vi "Simple Move.vi"(8 "error in (no error)":errorcluster, 10 "Move Data cluster":T1, 11 "Motions in":refnum<class "Motions.lvclass">) -> (0 "error out":errorcluster, 3 "Motions out":refnum<class "Motions.lvclass">)   [LabVIEW 2016, in "Hardware.lvlib" / "Motions.lvlib" / "Motions.lvclass"]
uses:
  <userlib>/Common Components/Hardware/Abstract System/Motions/Motions/Motions.lvclass
  <userlib>/Common Components/Hardware/Abstract System/Motions/Motions/Data_Move.ctl
  <userlib>/Common Components/Hardware/Abstract System/Motions/Motions/Motions.lvclass/Motions.ctl
  <userlib>/Common Components/Hardware/Motor/Motor/Motor.lvclass
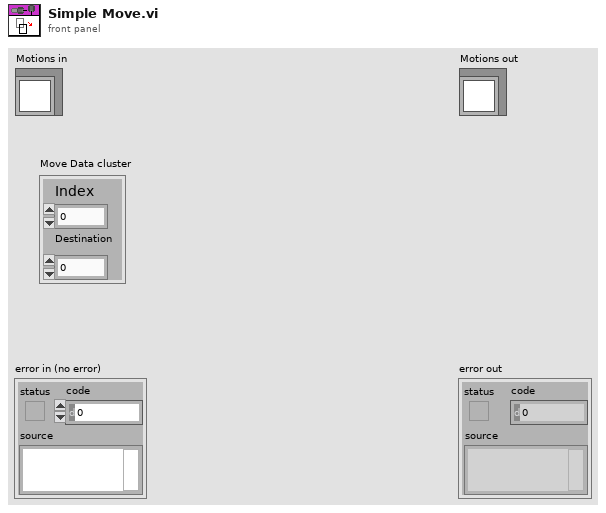
[diagram p1: front panel]
types:
  T1 = typedef "Hardware.lvlib/Motions.lvlib/Motions.lvclass/Data_Move.ctl" = cluster{"Index":i32, "Destination":dbl}
  T2 = typedef "Hardware.lvlib/Motions.lvlib/Motions.lvclass/Motor States.ctl" = cluster{"Connected":bool, "Enabled":bool, "Moving Status":bool, "Soft Moving Status":bool, "Current Pos":dbl, "Target Pos":dbl, "Moving Dir (-1, 0, 1)":i32, "Error Status":bool, "Hard Limit+":bool, "Hard Limit-":bool, "Soft Limit+":bool, "Soft Limit-":bool, "History Dst Stack":refnum<queue>, "Motion Status":bool, "Motion TriggerAction Obj":refnum<class "TriggerAction Q.lvclass">}
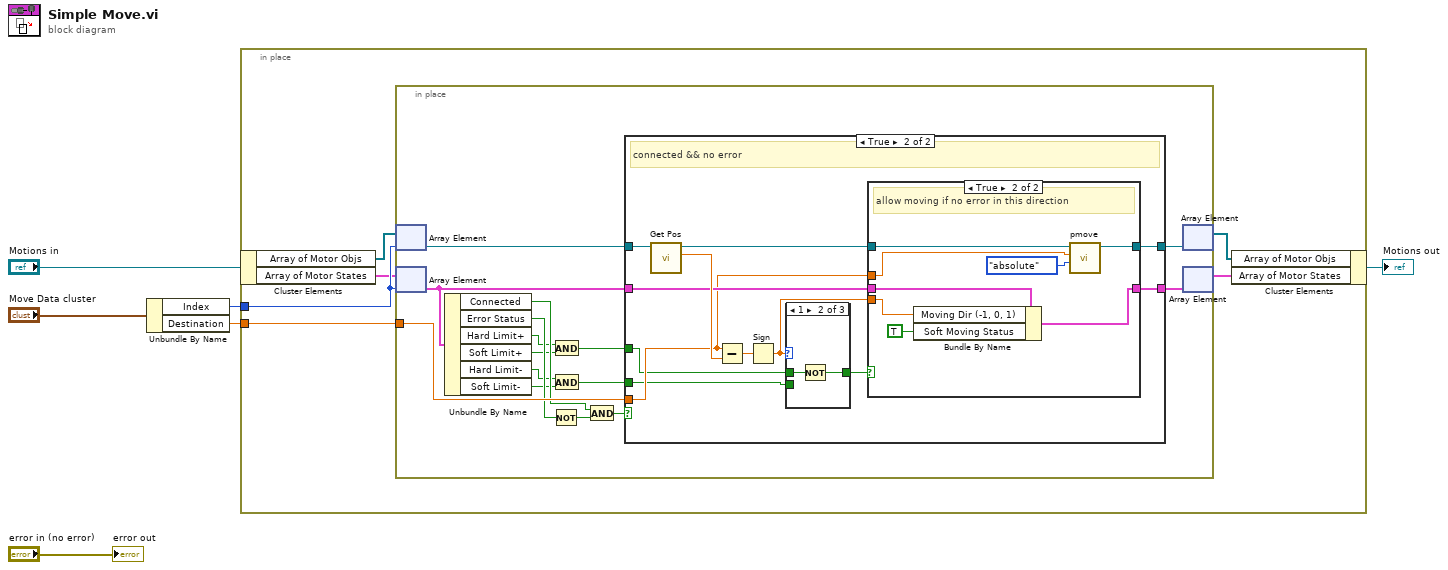
[diagram p0: block diagram]
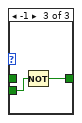
[diagram p4: hidden frame]
diagram:
  n1 = Unbundle By Name("Move Data cluster") -> ("Index"=w2:i32, "Destination"=w1:dbl)
  n2 = in-place {
    in-place-border: w2 -> [w9]
    in-place-border: w1 -> [w10]
    n3 = in-place-cluster #1("Motions in") -> ("Array of Motor Objs"=w12:refnum<class "Motor.lvclass">[], "Array of Motor States"=w8:T2[])
    n4 = in-place {
      in-place-border: w10 -> [w26]
      n5 = in-place-array #2(w12, w9) -> (w27:refnum<class "Motor.lvclass">)
      n6 = in-place-array #3(w8, w9) -> (w25:T2)
      n7 = Unbundle By Name(w25) -> ("Connected"=w23:bool, "Error Status"=w22:bool, "Hard Limit+"=w18:bool, "Soft Limit+"=w17:bool, "Hard Limit-"=w16:bool, "Soft Limit-"=w15:bool)
      n8 = Not(x=w22) -> (.not. x?=w21:bool)
      n9 = And(x=w18, y=w17) -> (x .and. y?=w14:bool)
      n10 = And(x=w16, y=w15) -> (x .and. y?=w13:bool)
      n11 = And(x=w23, y=w21) -> (x .and. y?=w20:bool)
      n12 = case shown="True" w20 {
        tunnel: w27 -> [w28 w34]
        tunnel: w26 -> [_ w35]
        tunnel: w25 -> [w29 w39]
        tunnel: [w29 w38] -> w24
        tunnel: [w28 w36] -> w19
        tunnel: w14 -> [_ w31]
        tunnel: w13 -> [_ w30]
        frame False {
        }
        frame True {
          # "connected && no error"
          n13 = call <userlib>:"Get Pos.vi"("Motor in"=w34) -> ("Position in unit mode (backend)"=w40:dbl, "Motor out"=w37:refnum<class "Motor.lvclass">)  [unwired: 7 in, 2 out]
          n14 = Subtract(x=w35, y=w40) -> (x-y=w41:dbl)
          n15 = Sign(1:w41) -> (0:w33:dbl)
          n16 = case shown="1" w33 {
            tunnel: [_ w42 w44] -> w32
            tunnel: w31 -> [_ w43 _]
            tunnel: w30 -> [_ _ w45]
            frame 0, Default {
            }
            frame 1 {
              n17 = Not(x=w43) -> (.not. x?=w42:bool)
            }
            frame -1 {
              n18 = Not(x=w45) -> (.not. x?=w44:bool)
            }
          }
          n19 = case shown="True" w32 {
            tunnel: w33 -> [_ w55]
            tunnel: w39 -> [w46 w54]
            tunnel: [w46 w53] -> w38
            tunnel: w37 -> [w47 w52]
            tunnel: [w47 w51] -> w36
            tunnel: w35 -> [_ w49]
            frame False {
            }
            frame True {
              # "allow moving if no error in this direction"
              n20 = Bundle By Name(cluster=w54, "Moving Dir (-1, 0, 1)"=w55, "Soft Moving Status"=TRUE) -> (w53:T2)
              n21 = call <userlib>:"pmove.vi"("mode (0: rel; 1: abs)"=enum16{"relative", "absolute"}."absolute", "distance in unit mode"=w49, "Motor in"=w52) -> ("Motor out"=w51:refnum<class "Motor.lvclass">)  [unwired: 7 in, 1 out]
            }
          }
        }
      }
      n22 = in-place-array #2(w19) -> (w11:refnum<class "Motor.lvclass">[])  [unwired: 1 out]
      n23 = in-place-array #3(w24) -> (w7:T2[])  [unwired: 1 out]
    }
    n24 = in-place-cluster #1("Array of Motor Objs"=w11, "Array of Motor States"=w7) -> (→"Motions out":refnum<class "Motions.lvclass">)
  }
  "error out" <- "error in (no error)"
